vi "Change Plot Visibility.vi"(0 "Data in":T1, 5 "Display State":T3, 9 "panel":refnum<vi>) -> (4 "Data out":T1, 15 "error out":errorcluster)   [LabVIEW 2015, in "Interactive Graph.xctl"]
uses:
  Interactive Graph.xctl
  State.vi
  Persistent.ctl
  Plot.ctl
  EPhys/LV Source/Work Panel VIs/Typedefs/EPhysWork-Label Position.ctl
  Events.ctl
  Selection.ctl
  XRange.ctl
  YScale.ctl
  Cursor.ctl
  Data.vi
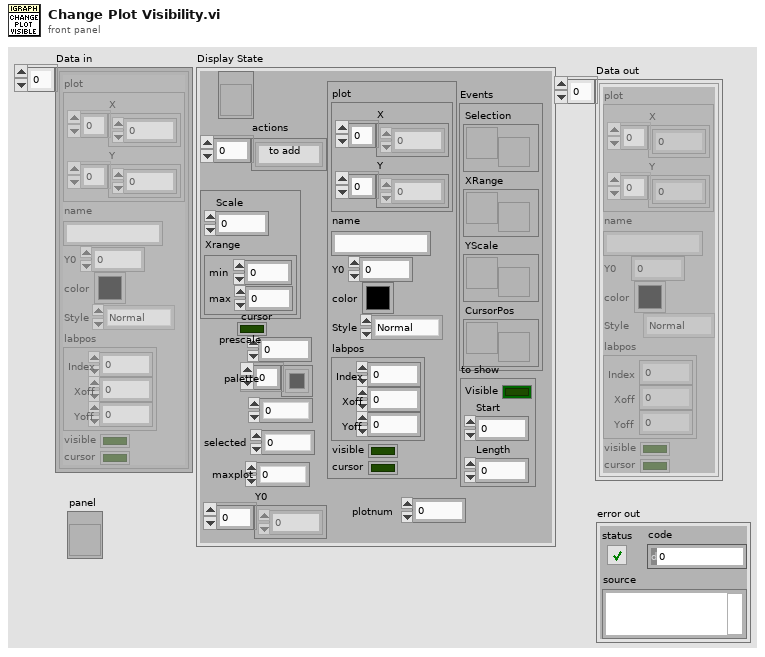
[diagram p1: front panel]
types:
  T1 = typedef "Interactive Graph.xctl/Data.vi" = cluster{"plot":cluster{"X":dbl[], "Y":dbl[]}, "name":string, "Y0":dbl, "color":u32, "Style":enum16{"Normal", "Highlight", "Shadow"}, "labpos":T2, "visible":bool, "cursor":bool}[]
  T2 = typedef "EPhysWork-Label Position.ctl" = cluster{"Index":i32, "Xoff":dbl, "Yoff":dbl}
  T3 = typedef "Interactive Graph.xctl/State.vi" = cluster{"ref":refnum<vi>, "actions":string[], "Persist":T4, "cursor":bool, "prescale":dbl, "palette":u32[], "colIndex":i32, "to add":T5, "Events":T6, "selected":i32, "to show":cluster{"Visible":bool, "Start":i32, "Length":i32}, "maxplot":i32, "Y0":dbl[], "plotnum":i32}
  T4 = typedef "Interactive Graph.xctl/Persistent.ctl" = cluster{"Scale":dbl, "Xrange":cluster{"min":dbl, "max":dbl}}
  T5 = typedef "Interactive Graph.xctl/Plot.ctl" = cluster{"plot":cluster{"X":dbl[], "Y":dbl[]}, "name":string, "Y0":dbl, "color":u32, "Style":enum16{"Normal", "Highlight", "Shadow"}, "labpos":T2, "visible":bool, "cursor":bool}
  T6 = typedef "Interactive Graph.xctl/Events.ctl" = cluster{"Selection":refnum<user-event>, "XRange":refnum<user-event>, "YScale":refnum<user-event>, "CursorPos":refnum<user-event>}
  T7 = typedef "LVAnnotationListTypeDef.ctl" = cluster{"Name":string, "Color":u32, "Style":u8, "Point Style":u8, "Name Visible":bool, "Allow Drag":bool, "Annotation Mode":u32, "Plot":i32, "Index":i32, "Position":cluster{"X":dbl, "Y":dbl}, "X Scale":u32, "Y Scale":u32, "Show Arrow":bool, "Lock Name":bool, "Plot Area":i32, "Label Offset":cluster{"X":dbl, "Y":dbl}}[]
  T8 = cluster{"Name":string, "Color":u32, "Style":u8, "Point Style":u8, "Name Visible":bool, "Allow Drag":bool, "Annotation Mode":u32, "Plot":i32, "Index":i32, "Position":cluster{"X":dbl, "Y":dbl}, "X Scale":u32, "Y Scale":u32, "Show Arrow":bool, "Lock Name":bool, "Plot Area":i32, "Label Offset":cluster{"X":dbl, "Y":dbl}}
  T9 = cluster{"plot":cluster{"X":dbl[], "Y":dbl[]}, "name":string, "Y0":dbl, "color":u32, "Style":enum16{"Normal", "Highlight", "Shadow"}, "labpos":T2, "visible":bool, "cursor":bool}
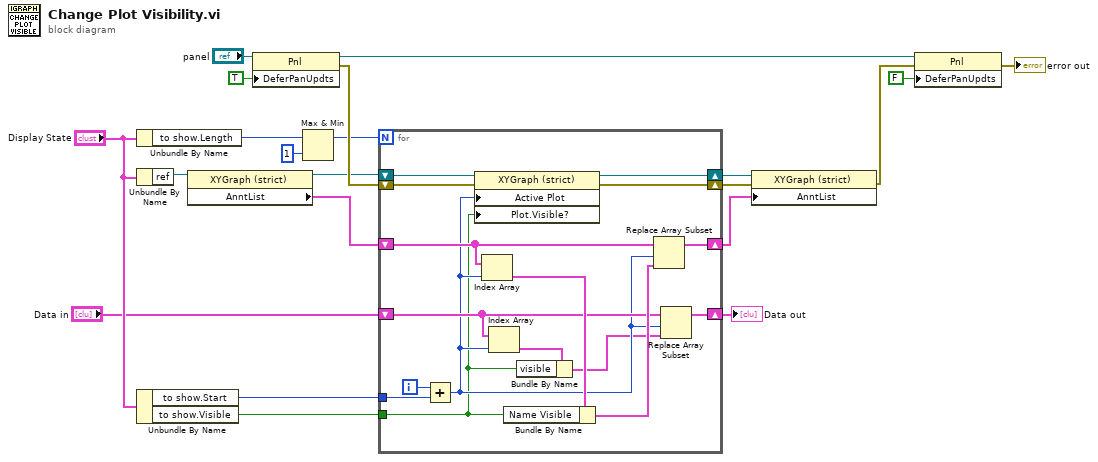
[diagram p0: block diagram]
diagram:
  n1 = Unbundle By Name("Display State") -> ("to show.Length"=w12:i32)
  n2 = Unbundle By Name("Display State") -> ("ref"=w8:refnum<vi>)
  n3 = Unbundle By Name("Display State") -> ("to show.Start"=w10:i32, "to show.Visible"=w14:bool)
  n4 = property class="XYGraph (strict)"(reference=w8) -> (reference out=w13:refnum<vi>, "AnntList"=w7:T7)  [unwired: 1 in, 1 out]
  n5 = property class="Pnl"(reference="panel", "DeferPanUpdts"=TRUE ("Defer Panel Updates")) -> (reference out=w17:refnum<vi>, error out=w21:errorcluster)  [unwired: 1 in]
  n6 = Max & Min(x=w12, y=1) -> (max(x,y)=w15:i32)  [unwired: 1 out]
  n7 = for {
    N: w15 -> [_]
    shift-right: [w36] -> w5
    shift-left: w21 -> [w35]
    tunnel: w14 -> [w22]
    shift-right: [w31] -> w6
    shift-left: w13 -> [w37]
    tunnel: w10 -> [w33]
    shift-right: [w28] -> w4
    shift-left: w7 -> [w30]
    shift-right: [w27] -> w1
    shift-left: "Data in" -> [w26]
    i -> [w34]
    n8 = Add(x=w34, y=w33) -> (x+y=w24:i32)
    n9 = property class="XYGraph (strict)"(reference=w37, error in=w35, "Active Plot"=w24, "Plot.Visible?"=w22) -> (reference out=w31:refnum<vi>, error out=w36:errorcluster)
    n10 = Index Array(array=w30, index=w24) -> (element=w32:T8)
    n11 = Index Array(array=w26, index=w24) -> (element=w25:T9)
    n12 = Bundle By Name(cluster=w32, "Name Visible"=w22) -> (w29:T8)
    n13 = Bundle By Name(cluster=w25, "visible"=w22) -> (w23:T9)
    n14 = Replace Array Subset(array=w30, new element=w29, index=w24) -> (w28:T7)
    n15 = Replace Array Subset(array=w26, new element=w23, index=w24) -> (w27:T1)
  }
  "Data out" <- w1
  n16 = property class="XYGraph (strict)"(reference=w6, error in=w5, "AnntList"=w4) -> (error out=w3:errorcluster)  [unwired: 1 out]
  n17 = property class="Pnl"(reference=w17, error in=w3, "DeferPanUpdts"=FALSE ("Defer Panel Updates")) -> (error out=→"error out":errorcluster)  [unwired: 1 out]
